vi "Populate Actual Values.vi"(8 "error in":errorcluster, 11 "UI Actor in":refnum<class "UI Actor.lvclass">) -> (0 "error out":errorcluster, 3 "UI Actor out":refnum<class "UI Actor.lvclass">)   [LabVIEW 2024, in "UI Actor.lvlib" / "UI Actor.lvclass"]
uses:
  UI Actor.lvclass
  UI Actor.lvclass/UI Actor.ctl
  Core/EDS/EDS.lvclass/EDS.ctl
  Core/EDS/EDS.lvclass
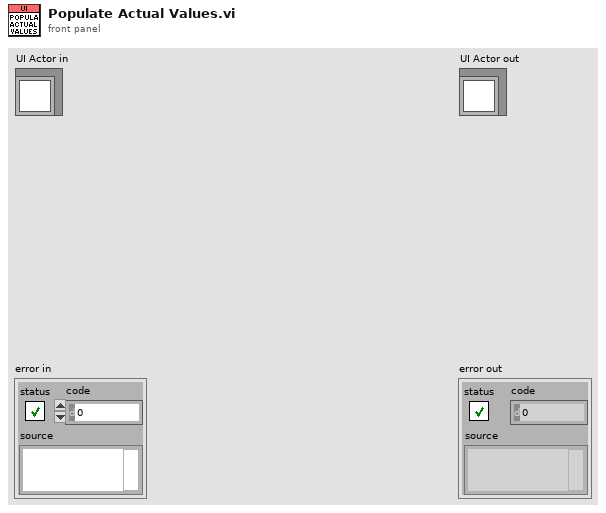
[diagram p1: front panel]
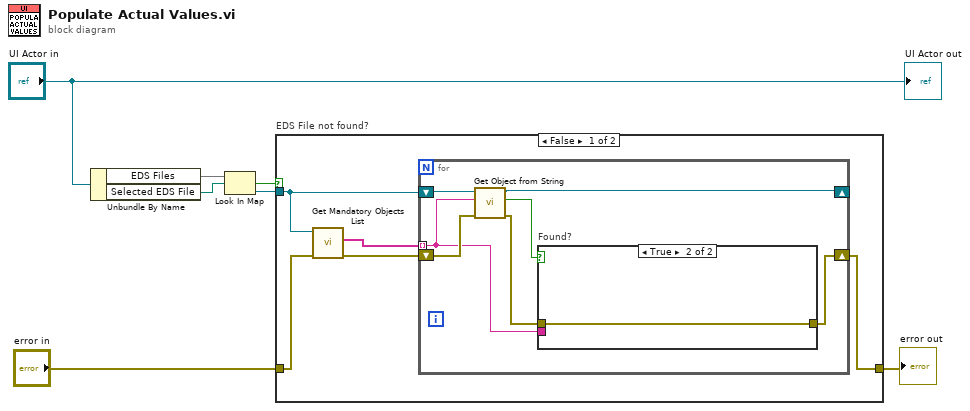
[diagram p0: block diagram]
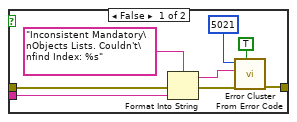
[diagram p2: hidden frame]
diagram:
  n1 = Unbundle By Name("UI Actor in") -> ("EDS Files"=w7:map{path, refnum<class "EDS.lvclass">}, "Selected EDS File"=w6:path)
  n2 = Look In Map(map=w7, key=w6) -> (key not found?=w4:bool, value=w3:refnum<class "EDS.lvclass">)  [unwired: 1 in]
  n3 = case "EDS File not found?" shown="False" w4 {
    tunnel: w3 -> [w8 _]
    tunnel: "error in" -> [w9 w29]
    tunnel: [w10 w29] -> w1
    frame False {
      n4 = call "Get Mandatory Objects List.vi"("error in"=w9, "EDS in"=w8) -> ("error out"=w11:errorcluster, "Objects List"=w12:string[])  [unwired: 7 in, 1 out]
      n5 = for {
        tunnel: w12 -> [w15] mode=indexing
        shift-right: [w17] -> w10
        shift-left: w11 -> [w19]
        shift-right: [w18] -> _
        shift-left: w8 -> [w13]
        n6 = call "Get Object from String.vi"("error in"=w19, "Index"=w15, "EDS in"=w13) -> ("error out"=w16:errorcluster, "Found?"=w14:bool, "EDS out"=w18:refnum<class "EDS.lvclass">)  [unwired: 5 in, 1 out]
        n7 = case "Found?" shown="True" w14 {
          tunnel: [w27 w28] -> w17
          tunnel: w16 -> [w23 w28]
          tunnel: w15 -> [w20 _]
          frame False {
            n8 = Format Into String(format string="Inconsistent Mandatory\nObjects Lists. Couldn't\nfind Index: %s" ("error message (\"\")"), error in=w23, w20) -> (resulting string=w24:string, error out=w22:errorcluster)  [unwired: 1 in]
            n9 = call <vilib>:"Error Cluster From Error Code.vi"("show call chain? (False)"=TRUE, "error in (no error)"=w22, "error message (\"\")"=w24, "error code (0)"=5021) -> ("error out"=w27:errorcluster)  [unwired: 5 in]
          }
          frame True {
          }
        }
      }
    }
    frame True {
    }
  }
  "error out" <- w1
  "UI Actor out" <- "UI Actor in"
